vi "ScanListParse.vi"(10 "ApplicationNumberOfWeldChannels":i32, 11 "Input":string="SCANALL") -> (3 "Output":string[](array[string]))   [LabVIEW 2019]
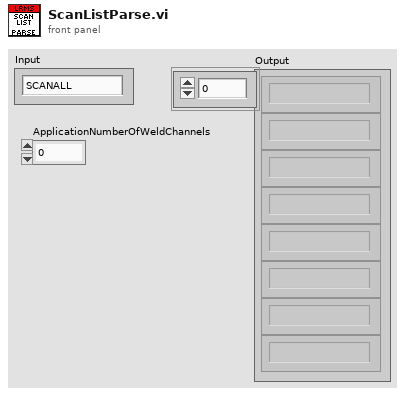
[diagram p1: front panel]
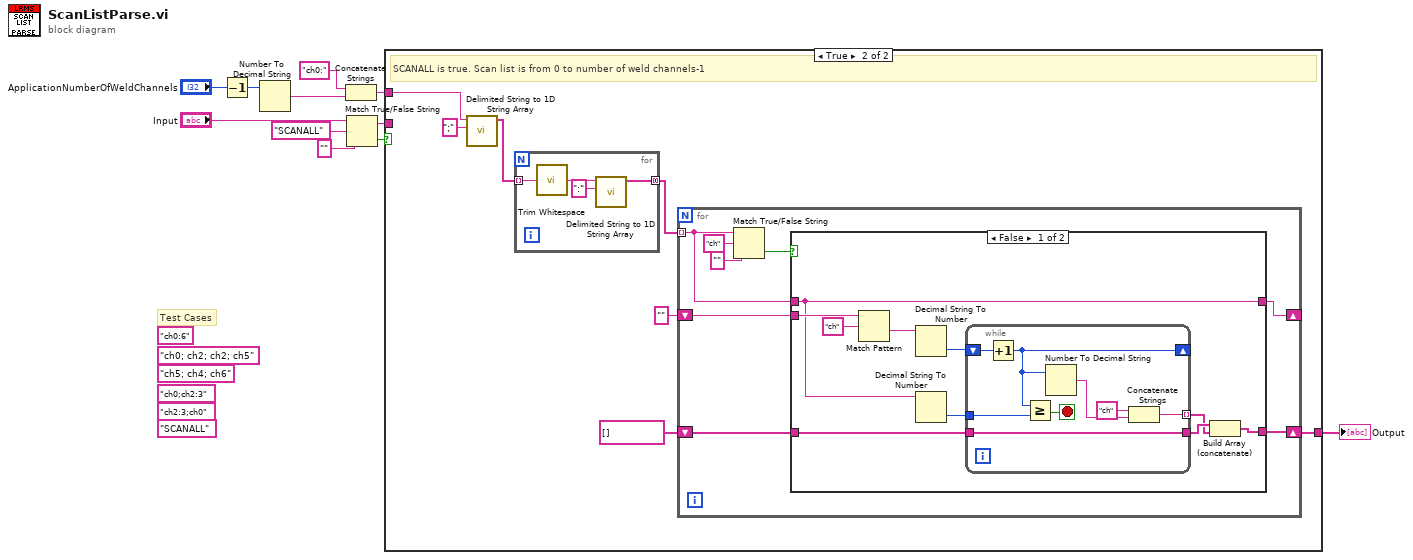
[diagram p0: block diagram]
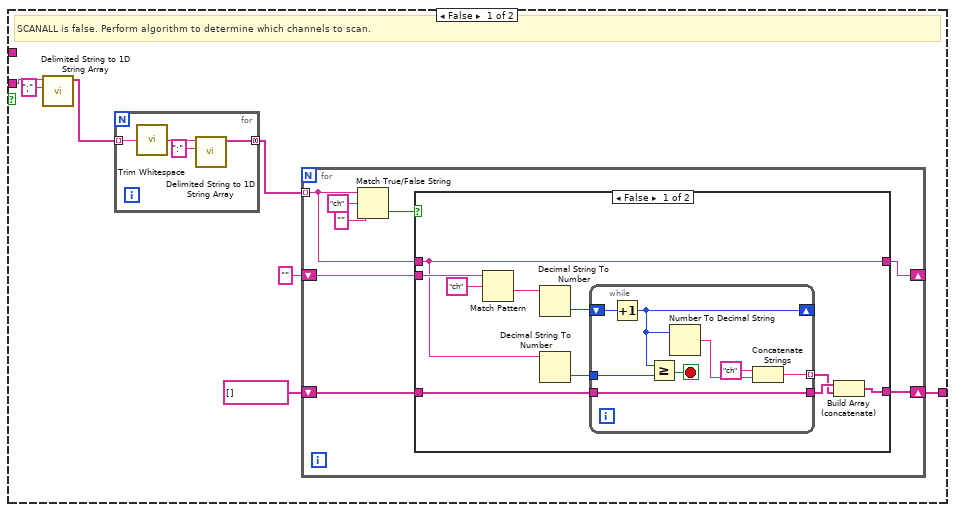
[diagram p2: hidden frame]
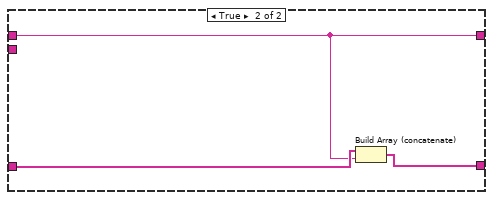
[diagram p3: hidden frame]
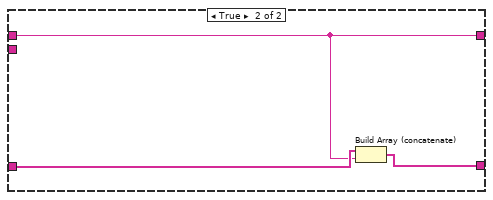
[diagram p4: hidden frame]
diagram:
  (unwired) "SCANALL" ("Input 2")
  (unwired) "ch5; ch4; ch6"
  (unwired) "ch0; ch2; ch2; ch5"
  (unwired) "ch0:6"
  (unwired) "ch2:3;ch0"
  (unwired) "ch0;ch2:3"
  # "Test Cases"
  n1 = Decrement(x="ApplicationNumberOfWeldChannels") -> (x-1=w4:i32)
  n2 = Number To Decimal String(number=w4) -> (decimal integer string=w2:string)  [unwired: 1 in]
  n3 = Concatenate Strings("ch0:", w2) -> (w1:string)
  n4 = Match True/False String(2:"" ("false string"), 3:"SCANALL" ("true string"), 4:"Input") -> (0:w7:bool, 1:w8:string)
  n5 = case shown="True" w7 {
    tunnel: [w13 w53] -> w11
    tunnel: w8 -> [w12 _]
    tunnel: w1 -> [_ w52]
    frame False {
      # "SCANALL is false. Perform algorithm to determine which channels to scan."
      n6 = call <vilib>:"Delimited String to 1D String Array.vi"("delimiter"=";", "delimited string"=w12) -> ("string array"=w17:string[])  [unwired: 9 in]
      n7 = for {
        tunnel: w17 -> [w50] mode=indexing
        tunnel: [w49] -> w16 mode=concatenating
        n8 = call <vilib>:"Trim Whitespace.vi"("string"=w50) -> ("trimmed string"=w48:string)  [unwired: 1 in]
        n9 = call <vilib>:"Delimited String to 1D String Array.vi"("delimiter"=":", "delimited string"=w48) -> ("string array"=w49:string[])  [unwired: 9 in]
      }
      n10 = for {
        tunnel: w16 -> [w23] mode=indexing
        shift-right: [w20] -> _
        shift-left: "" ("String") -> [w22]
        shift-right: [w19] -> w13
        shift-left: string[] [] -> [w21]
        n11 = Match True/False String(2:"" ("false string"), 3:"ch" ("true string"), 4:w23) -> (0:w24:bool)  [unwired: 1 out]
        n12 = case shown="False" w24 {
          tunnel: w23 -> [w33 w45]
          tunnel: [w33 w45] -> w20
          tunnel: w22 -> [w35 _]
          tunnel: [w29 w47] -> w19
          tunnel: w21 -> [w30 w46]
          frame False {
            n13 = Match Pattern(string=w35, regular expression="ch") -> (after substring=w34:string)  [unwired: 1 in, 3 out]
            n14 = Decimal String To Number(string=w34) -> (number=w31:i32)  [unwired: 2 in, 1 out]
            n15 = Decimal String To Number(string=w33) -> (number=w32:i32)  [unwired: 2 in, 1 out]
            n16 = while {
              tunnel: [w41] -> w27 mode=indexing
              tunnel: w30 -> [w37]
              shift-right: [w38] -> _
              shift-left: w31 -> [w39]
              tunnel: w32 -> [w40]
              tunnel: [w37] -> w28
              stop <- w44 stop-if-true
              n17 = Increment(x=w39) -> (x+1=w38:i32)
              n18 = Greater Or Equal?(x=w38, y=w40) -> (x >= y?=w44:bool)
              n19 = Number To Decimal String(number=w38) -> (decimal integer string=w42:string)  [unwired: 1 in]
              n20 = Concatenate Strings("ch" ("element"), w42) -> (w41:string)
            }
            n21 = Build Array (concatenate)(w28, w27) -> (w29:string[])
          }
          frame True {
            n22 = Build Array (concatenate)(w46, w45) -> (w47:string[])
          }
        }
      }
    }
    frame True {
      # "SCANALL is true. Scan list is from 0 to number of weld channels-1"
      n23 = call <vilib>:"Delimited String to 1D String Array.vi"("delimiter"=";", "delimited string"=w52) -> ("string array"=w57:string[])  [unwired: 9 in]
      n24 = for {
        tunnel: w57 -> [w90] mode=indexing
        tunnel: [w89] -> w56 mode=concatenating
        n25 = call <vilib>:"Trim Whitespace.vi"("string"=w90) -> ("trimmed string"=w88:string)  [unwired: 1 in]
        n26 = call <vilib>:"Delimited String to 1D String Array.vi"("delimiter"=":", "delimited string"=w88) -> ("string array"=w89:string[])  [unwired: 9 in]
      }
      n27 = for {
        tunnel: w56 -> [w63] mode=indexing
        shift-right: [w60] -> _
        shift-left: "" ("String") -> [w62]
        shift-right: [w59] -> w53
        shift-left: string[] [] -> [w61]
        n28 = Match True/False String(2:"" ("false string"), 3:"ch" ("true string"), 4:w63) -> (0:w64:bool)  [unwired: 1 out]
        n29 = case shown="False" w64 {
          tunnel: w63 -> [w73 w85]
          tunnel: [w73 w85] -> w60
          tunnel: w62 -> [w75 _]
          tunnel: [w69 w87] -> w59
          tunnel: w61 -> [w70 w86]
          frame False {
            n30 = Match Pattern(string=w75, regular expression="ch") -> (after substring=w74:string)  [unwired: 1 in, 3 out]
            n31 = Decimal String To Number(string=w74) -> (number=w71:i32)  [unwired: 2 in, 1 out]
            n32 = Decimal String To Number(string=w73) -> (number=w72:i32)  [unwired: 2 in, 1 out]
            n33 = while {
              tunnel: [w81] -> w67 mode=indexing
              tunnel: w70 -> [w77]
              shift-right: [w78] -> _
              shift-left: w71 -> [w79]
              tunnel: w72 -> [w80]
              tunnel: [w77] -> w68
              stop <- w84 stop-if-true
              n34 = Increment(x=w79) -> (x+1=w78:i32)
              n35 = Greater Or Equal?(x=w78, y=w80) -> (x >= y?=w84:bool)
              n36 = Number To Decimal String(number=w78) -> (decimal integer string=w82:string)  [unwired: 1 in]
              n37 = Concatenate Strings("ch" ("element"), w82) -> (w81:string)
            }
            n38 = Build Array (concatenate)(w68, w67) -> (w69:string[])
          }
          frame True {
            n39 = Build Array (concatenate)(w86, w85) -> (w87:string[])
          }
        }
      }
    }
  }
  "Output" <- w11
